vi "ICNC Read EEPROM.vi"(8 "error in (no error)":errorcluster caption="entrée d'erreur (pas d'erreur)", 9 "Value":string, 10 "Length":u32, 11 "StartAdress":u32) -> (0 "error out":errorcluster caption="sortie d'erreur", 1 "Value out":string, 3 "function return":u32)   [LabVIEW 2012, in "ICNC2.lvlib"]
doc: "DWORD ICNC_ReadEEPROM( DWORD StartAdress,\n DWORD Length,\n BYTE* Value);"
uses:
  <userlib>/ICNC/ICNC2.lvlib
  <userlib>/ICNC/ICNC2.dll
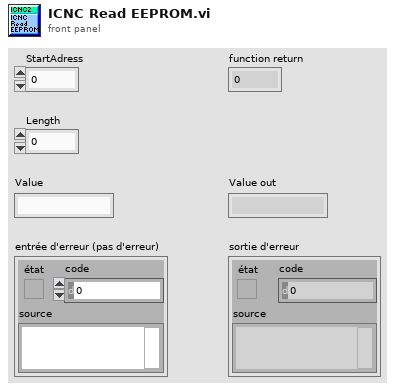
[diagram p1: front panel]
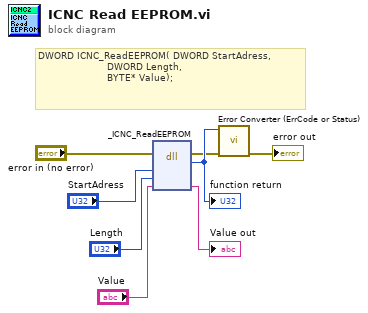
[diagram p0: block diagram]
diagram:
  # "DWORD ICNC_ReadEEPROM( DWORD StartAdress,\n                       DWORD Length,\n                       BYTE* Value);"
  n1 = dll-call lib="C:/Program Files (x86)/National Instruments/LabVIEW 2012/user.lib/ICNC/ICNC2.*" fn="_ICNC_ReadEEPROM"(error in="error in (no error)", "StartAdress"="StartAdress", "Length"="Length", "Value"="Value") -> (error out=w2:errorcluster, w8:u32, "Value"=→"Value out":string)  [unwired: 4 in, 1 out]
  "function return" <- w8
  n2 = call <userlib>:"Error Converter (ErrCode or Status).vi"("error in (no error)"=w2, "error code"=w8) -> ("error out"=→"error out":errorcluster)  [unwired: 9 in]
